vi "Update Measurement Details.vi"(8 "error in":errorcluster, 9 "measurement service description":string, 10 "measurement service name":string, 11 "project ref":refnum<vi>) -> (0 "error out":errorcluster, 3 "project ref out":refnum<vi>)   [LabVIEW 2021, in "MeasurementService Editor.lvlib"]
uses:
  MeasurementService Editor.lvlib
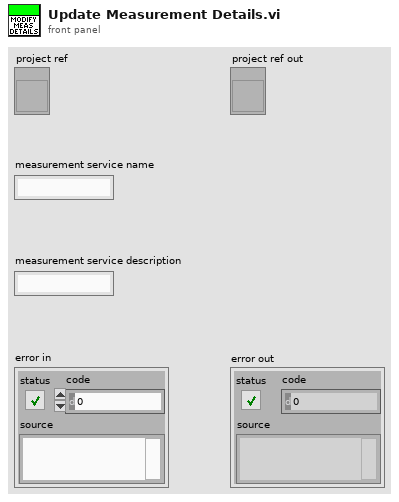
[diagram p1: front panel]
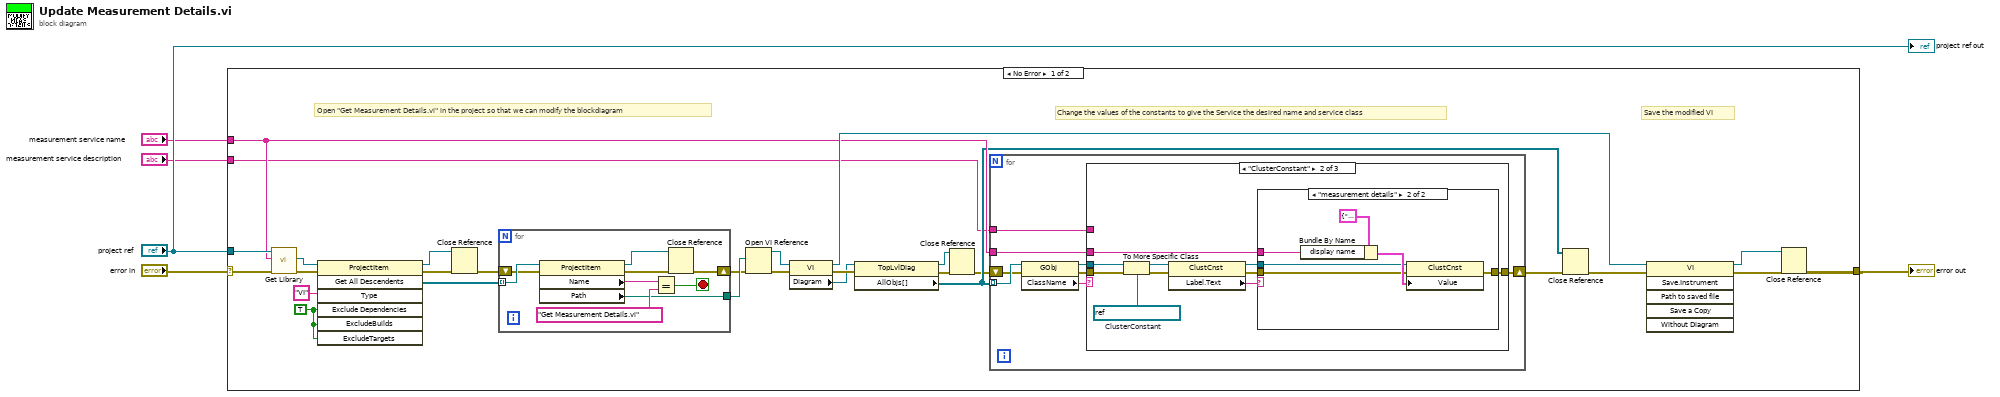
[diagram p0: block diagram]
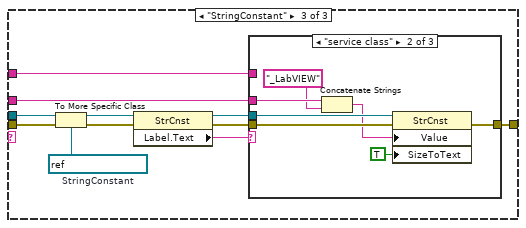
[diagram p4: hidden frame]
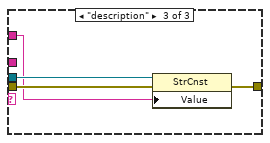
[diagram p6: hidden frame]
diagram:
  n1 = case shown="No Error" "error in" {
    selector: "error in" -> [w21 w92]
    tunnel: "project ref" -> [w20 _]
    tunnel: [w31 w92] -> w3
    tunnel: "measurement service name" -> [w14 _]
    tunnel: "measurement service description" -> [w6 _]
    frame No Error {
      w33 = TRUE ("ExcludeDependencies")
      # "Save the modified VI"
      # "Open \"Get Measurement Details.vi\" in the project so that we can modify the blockdiagram"
      # "Change the values of the constants to give the Service the desired name and service class"
      n2 = call "Get Library.vi"("error in (no error)"=w21, "library name"=w14, "project ref"=w20) -> ("error out"=w19:errorcluster, "library item"=w18:refnum<vi>)  [unwired: 5 in, 2 out]
      n3 = invoke class="ProjectItem" method="Get All Descendents"(reference=w18, error in=w19, "Type"="VI", "Exclude Dependencies"=w33, "ExcludeBuilds"=w33, "ExcludeTargets"=w33) -> (reference out=w15:refnum<vi>, error out=w17:errorcluster, "All Descendents"=w13:refnum<vi>[])  [unwired: 1 in, 4 out]
      n4 = Close Reference(reference=w15, error in (no error)=w17) -> (error out=w16:errorcluster)
      n5 = for {
        tunnel: w13 -> [w91] mode=indexing
        shift-right: [w84] -> w11
        shift-left: w16 -> [w88]
        tunnel: [w86] -> w12
        stop <- w87 stop-if-true
        n6 = property class="ProjectItem"(reference=w91, error in=w88) -> (reference out=w83:refnum<vi>, error out=w85:errorcluster, "Name"=w89:string, "Path"=w86:path)
        n7 = Equal?(x=w89, y="Get Measurement Details.vi") -> (x = y?=w87:bool)
        n8 = Close Reference(reference=w83, error in (no error)=w85) -> (error out=w84:errorcluster)
      }
      n9 = Open VI Reference(vi path=w12, error in (no error)=w11) -> (vi reference=w28:refnum<vi>, error out=w26:errorcluster)  [unwired: 4 in]
      n10 = property class="VI"(reference=w28, error in=w26) -> (reference out=w24:refnum<vi>, error out=w27:errorcluster, "Diagram"=w25:refnum<vi>)
      n11 = property class="TopLvlDiag"(reference=w25, error in=w27) -> (reference out=w7:refnum<vi>, error out=w9:errorcluster, "AllObjs[]"=w10:refnum<vi>[])
      n12 = Close Reference(reference=w7, error in (no error)=w9) -> (error out=w8:errorcluster)
      n13 = for {
        tunnel: w10 -> [w41] mode=indexing
        shift-right: [w35] -> w23
        shift-left: w8 -> [w40]
        tunnel: w14 -> [w36]
        tunnel: w6 -> [w34]
        n14 = property class="GObj"(reference=w41, error in=w40) -> (reference out=w38:refnum<vi>, error out=w37:errorcluster, "ClassName"=w39:string)
        n15 = case shown="\"ClusterConstant\"" w39 {
          tunnel: w38 -> [_ w51 w69]
          tunnel: w37 -> [w42 w50 w68]
          tunnel: w36 -> [_ w49 w61]
          tunnel: [w42 w48 w67] -> w35
          tunnel: w34 -> [_ _ w60]
          frame Default {
          }
          frame "ClusterConstant" {
            w52 = refnum<vi> refnum  # ClusterConstant
            n16 = To More Specific Class(target class=w52, reference=w51, error in=w50) -> (specific class reference=w47:refnum<vi>, error out=w46:errorcluster)
            n17 = property class="ClustCnst"(reference=w47, error in=w46) -> (reference out=w45:refnum<vi>, error out=w44:errorcluster, "Label.Text"=w43:string)
            n18 = case shown="\"measurement details\"" w43 {
              tunnel: w49 -> [_ w58]
              tunnel: [w53 w57] -> w48
              tunnel: w45 -> [_ w55]
              tunnel: w44 -> [w53 w54]
              frame Default {
              }
              frame "measurement details" {
                n19 = Bundle By Name(cluster=cluster{"display name":string, "version":string} {"display name"="Measurement Template", "version"="1.0.0"} ("ni_measurements_v1_MeasurementDetails"), "display name"=w58) -> (w56:cluster{"display name":string, "version":string})
                n20 = property class="ClustCnst"(reference=w55, error in=w54, "Value"=w56) -> (error out=w57:errorcluster)  [unwired: 1 out]
              }
            }
          }
          frame "StringConstant" {
            w70 = refnum<vi> refnum  # StringConstant
            n21 = To More Specific Class(target class=w70, reference=w69, error in=w68) -> (specific class reference=w66:refnum<vi>, error out=w65:errorcluster)
            n22 = property class="StrCnst"(reference=w66, error in=w65) -> (reference out=w63:refnum<vi>, error out=w62:errorcluster, "Label.Text"=w64:string)
            n23 = case shown="\"service class\"" w64 {
              tunnel: [w71 w78 w82] -> w67
              tunnel: w63 -> [_ w77 w81]
              tunnel: w62 -> [w71 w76 w80]
              tunnel: w61 -> [_ w75 _]
              tunnel: w60 -> [_ _ w79]
              frame Default {
              }
              frame "service class" {
                n24 = Concatenate Strings(w75, "_LabVIEW" ("string")) -> (w73:string)
                n25 = property class="StrCnst"(reference=w77, error in=w76, "Value"=w73, "SizeToText"=TRUE ("Size To Text?")) -> (error out=w78:errorcluster)  [unwired: 1 out]
              }
              frame "description" {
                n26 = property class="StrCnst"(reference=w81, error in=w80, "Value"=w79) -> (error out=w82:errorcluster)  [unwired: 1 out]
              }
            }
          }
        }
      }
      n27 = Close Reference(reference=w10, error in (no error)=w23) -> (error out=w22:errorcluster)
      n28 = invoke class="VI" method="Save.Instrument"(reference=w24, error in=w22) -> (reference out=w30:refnum<vi>, error out=w29:errorcluster)  [unwired: 4 in, 4 out]
      n29 = Close Reference(reference=w30, error in (no error)=w29) -> (error out=w31:errorcluster)
    }
    frame Error {
    }
  }
  "error out" <- w3
  "project ref out" <- "project ref"
